vi "RFH-test.vi"() -> ()   [LabVIEW 2020, in "RFH-Reflection_File_Handler.lvlib"]
uses:
  RFH-Reflection_File_Handler.lvlib
  RFH-common_data_format.ctl
panel:
  out "Common Format 4":T1
  out "Common Format 3":T1
  out "Common Format 2":T1
  out "Common Format":T1
  out "r140":bool
  out "libreVNA":bool
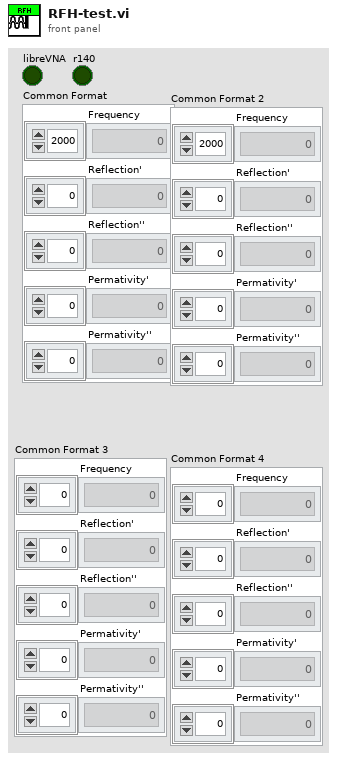
[diagram p1: front panel]
types:
  T1 = typedef "RFH-Reflection_File_Handler.lvlib/RFH-common_data_format.ctl" = cluster{"Frequency":dbl[], "Reflection'":dbl[], "Reflection''":dbl[], "Permativity'":dbl[], "Permativity''":dbl[]}
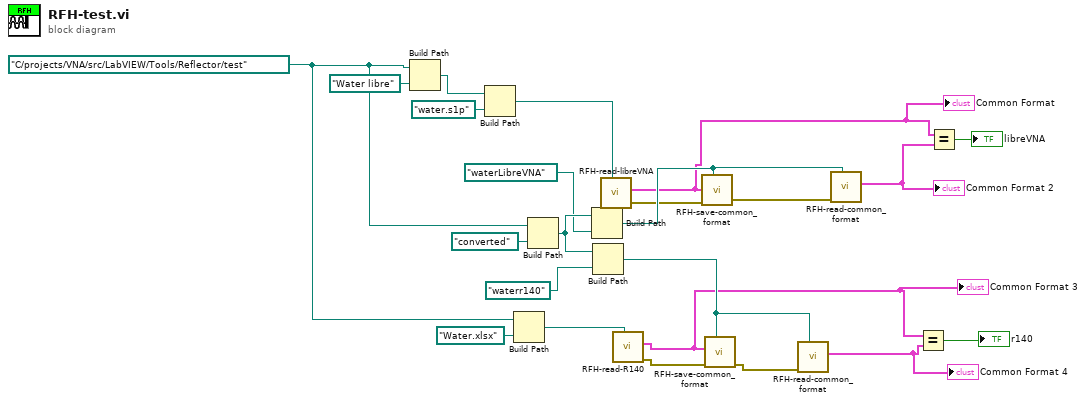
[diagram p0: block diagram]
diagram:
  w18 = path "C:/projects/VNA/src/LabVIEW/Tools/Reflector/test" ("file path (dialog if empty)")
  n1 = Build Path(base path=w18, name or relative path=path "Water libre") -> (appended path=w22:path)
  n2 = Build Path(base path=w22, name or relative path=path "water.s1p") -> (appended path=w17:path)
  n3 = Build Path(base path=w18, name or relative path=path "Water.xlsx") -> (appended path=w16:path)
  n4 = Build Path(base path=w18, name or relative path=path "converted") -> (appended path=w15:path)
  n5 = Build Path(base path=w15, name or relative path=path "waterLibreVNA") -> (appended path=w14:path)
  n6 = Build Path(base path=w15, name or relative path=path "waterr140") -> (appended path=w11:path)
  n7 = call "RFH-read-libreVNA.vi"("file path (dialog if empty)"=w17) -> ("error out"=w5:errorcluster, "Common Format"=w13:T1)  [unwired: 9 in]
  "Common Format" <- w13
  n8 = call "RFH-read-R140.vi"("file path (dialog if empty)"=w16) -> ("error out"=w4:errorcluster, "Common Format"=w2:T1)  [unwired: 8 in, 1 out]
  "Common Format 3" <- w2
  n9 = call "RFH-save-common_format.vi"("file path (use dialog)"=w14, "error in (no error)"=w5, "Common Format"=w13) -> ("error out"=w6:errorcluster)  [unwired: 8 in]
  n10 = call "RFH-save-common_format.vi"("file path (use dialog)"=w11, "error in (no error)"=w4, "Common Format"=w2) -> ("error out"=w3:errorcluster)  [unwired: 8 in]
  n11 = call "RFH-read-common_format.vi"("file path (dialog if empty)"=w11, "error in"=w3) -> ("Common Format"=w1:T1)  [unwired: 8 in, 1 out]
  "Common Format 4" <- w1
  n12 = call "RFH-read-common_format.vi"("file path (dialog if empty)"=w14, "error in"=w6) -> ("Common Format"=w12:T1)  [unwired: 8 in, 1 out]
  "Common Format 2" <- w12
  n13 = Equal?(x=w2, y=w1) -> (x = y?=→"r140":bool)
  n14 = Equal?(x=w13, y=w12) -> (x = y?=→"libreVNA":bool)
